vi "parse_serial_string.vi"(8 "Error In":errorcluster, 11 "Input String":string) -> (0 "Error Out":errorcluster, 1 "Load":dbl, 2 "Displacement":dbl, 3 "Time":dbl)   [LabVIEW 2021]
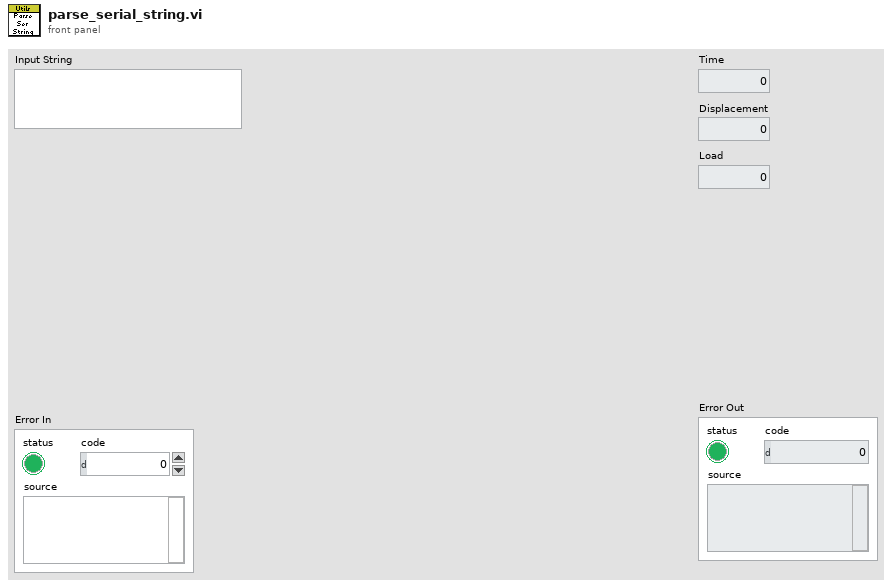
[diagram p1: front panel]
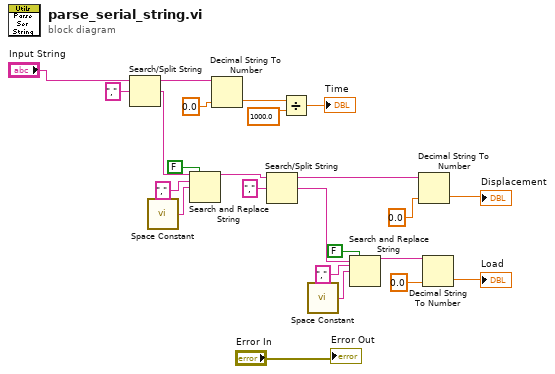
[diagram p0: block diagram]
diagram:
  n1 = Search/Split String(string="Input String", search string/char (-)=",") -> (substring before match=w23:string, match + rest of string=w3:string)  [unwired: 1 in, 1 out]
  n2 = call <vilib>:"Space Constant.vi"() -> ("String"=w15:string)
  n3 = Search and Replace String(replace all?=FALSE ("replace all? (F)"), input string=w3, search string=",", replace string=w15) -> (result string=w2:string)  [unwired: 4 in, 3 out]
  n4 = Decimal String To Number(string=w23, default (0L)=0.0) -> (number=w20:dbl)  [unwired: 1 in, 1 out]
  n5 = Search/Split String(string=w2, search string/char (-)=",") -> (substring before match=w1:string, match + rest of string=w8:string)  [unwired: 1 in, 1 out]
  n6 = Divide(x=w20, y=1000.0) -> (x/y=→"Time":dbl)
  n7 = call <vilib>:"Space Constant.vi"() -> ("String"=w10:string)
  n8 = Search and Replace String(replace all?=FALSE ("replace all? (F)"), input string=w8, search string=",", replace string=w10) -> (result string=w7:string)  [unwired: 4 in, 3 out]
  n9 = Decimal String To Number(string=w1, default (0L)=0.0) -> (number=→"Displacement":dbl)  [unwired: 1 in, 1 out]
  n10 = Decimal String To Number(string=w7, default (0L)=0.0) -> (number=→"Load":dbl)  [unwired: 1 in, 1 out]
  "Error Out" <- "Error In"
